vi "WaitMultiple.vi"(7 "wait option? (MoveDone)":i32(ring)=1 items=["InPosition", "MoveDone"], 8 "error in (no error)":errorcluster, 9 "timeout? (-1)":i32=-1, 10 "axis names":string[](array[string]), 11 "controller in":refnum<k24>) -> (0 "error out":errorcluster, 2 "completed":bool, 3 "controller out":refnum<k24>)   [LabVIEW 2013]
uses:
  C:/GEECS/Developers Version/source/Device Driver/AerotechStage/Sample Vis/Bin/Aerotech.Ensemble.dll
  Bin/Aerotech.Ensemble.dll
  C:/GEECS/Developers Version/source/Device Driver/AerotechStage/Sample Vis/Bin/Aerotech.Ensemble.LabVIEW.dll
  Bin/Aerotech.Ensemble.LabVIEW.dll
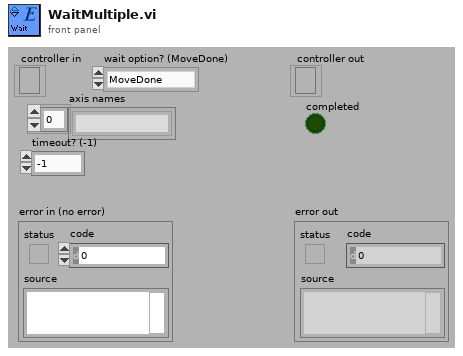
[diagram p1: front panel]
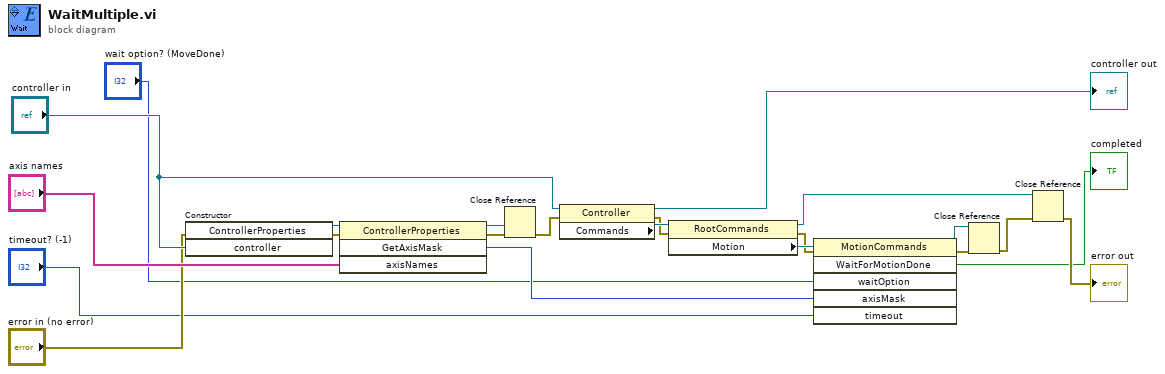
[diagram p0: block diagram]
diagram:
  n1 = constructor class="ControllerProperties"(error in="error in (no error)", "controller"="controller in") -> (reference out=w11:refnum<k24>, error out=w10:errorcluster)  [unwired: 2 in, 2 out]
  n2 = invoke class="ControllerProperties" method="GetAxisMask"(reference=w11, error in=w10, "axisNames"="axis names") -> (reference out=w8:refnum<k24>, error out=w9:errorcluster, "GetAxisMask"=w3:i32)  [unwired: 1 in, 1 out]
  n3 = Close Reference(reference=w8, error in (no error)=w9) -> (error out=w7:errorcluster)
  n4 = property class="Controller"(reference="controller in", error in=w7) -> (reference out=→"controller out":refnum<k24>, error out=w19:errorcluster, "Commands"=w21:refnum<k24>)
  n5 = property class="RootCommands"(reference=w21, error in=w19) -> (reference out=w13:refnum<k24>, error out=w18:errorcluster, "Motion"=w20:refnum<k24>)
  n6 = invoke class="MotionCommands" method="WaitForMotionDone"(reference=w20, error in=w18, "waitOption"="wait option? (MoveDone)", "axisMask"=w3, "timeout"="timeout? (-1)") -> (reference out=w14:refnum<k24>, error out=w17:errorcluster, "WaitForMotionDone"=→"completed":bool)  [unwired: 1 in, 3 out]
  n7 = Close Reference(reference=w14, error in (no error)=w17) -> (error out=w15:errorcluster)
  n8 = Close Reference(reference=w13, error in (no error)=w15) -> (error out=→"error out":errorcluster)
